vi "UIRef.vi"(8 "error in":errorcluster, 11 "ddds editor node in":refnum<class "dds editor node.lvclass">) -> (0 "error out":errorcluster, 2 "VI refnum":refnum<vi>, 3 "dds editor node out":refnum<class "dds editor node.lvclass">)   [LabVIEW 2020, in "DDS editor node.lvclass"]
uses:
  dds editor node.lvclass
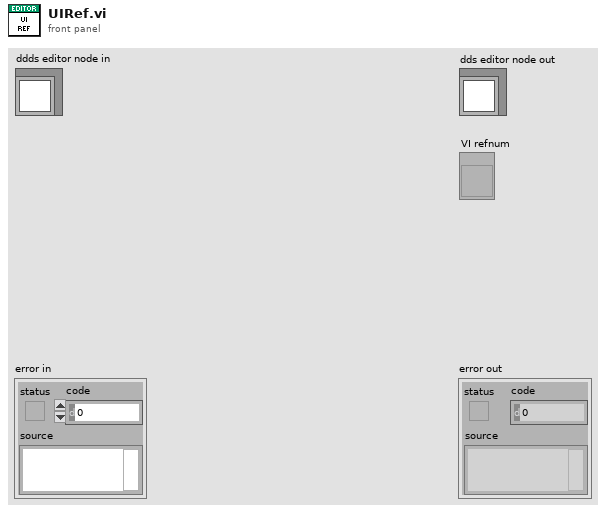
[diagram p1: front panel]
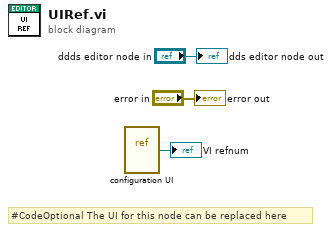
[diagram p0: block diagram]
diagram:
  # "#CodeOptional The UI for this node can be replaced here"
  n1 = vi-ref "configuration UI.vi"() -> (→"VI refnum":refnum<vi>)
  "error out" <- "error in"
  "dds editor node out" <- "ddds editor node in"
